vi "Ic Distribution_box.vi"(0 "device in":tag="Dev1", 1 "Scale factor":dbl=1.0, 2 "maximum value":dbl=5.0 format="%#_13g", 3 "Log Data":bool=TRUE, 5 "Trigger source":tag="/Dev1/PFI0", 7 "Current Read":tag="Dev1/ai2", 9 "Sample Rate":dbl=50.0 format="%.3p", 11 "error in no error":errorcluster, 12 "Points Number":i32=10000, 13 "Points per loop":i32=1000, 14 "minimum value":dbl format="%#_13g") -> (4 "Ic array":dbl[](array[numeric]), 15 "error out":errorcluster)   [LabVIEW 2021]
uses:
  <vilib>/DAQmx/read.llb/DAQmx Read (Analog 1D DBL 1Chan NSamp).vi
  <vilib>/DAQmx/create/channels.llb/DAQmx Create Channel (AI-Voltage-Basic).vi
  <vilib>/DAQmx/configure/timing.llb/DAQmx Timing (Sample Clock).vi
  <vilib>/DAQmx/miscellaneous.llb/DAQmx Fill In Error Info.vi
  Transport measurement/VIs/global.vi
  <vilib>/Analysis/NI_AALBase.lvlib
panel:
  out "millisecond timer value":u32=9828879
  in  "Tab Control":enum32{"AWG", "DAQ", "Curve", "Error"}(tab)=enum."Curve"
  in  "Sampling Frequency Hz":u64=10000000
  in  "End time S":dbl=0.005
  in  "Delay time S":dbl=0.3
  in  "Ramp time S":dbl=0.01
  in  "Amplitude V":dbl=5.0 format="%#_13g"
  in  "Channel Name":u16(ring)=1 items=["1"=1, "2"=2, "3"=3, "4"=4]
  in  "Update Wave":bool=TRUE
  in  "Use AWG":bool
  out "Points get":i32=10000
  in  "intervals":i32=100
  out "Histogram Graph":T1(graph)={"X Values"=[3.5826407117095322, 3.586252819563783, 3.589864927418034, 3.5934770352722847, 3.5970891431265355, 3.6007012509807863, 3.604313358835037, 3.607925466689288, 3.6115375745435387, 3.6151496823977896, 3.6187617902520404, 3.622373898106291, 3.625986005960542, 3.629598113814793, 3.6332102216690436, 3.6368223295232944, 3.6404344373775452, 3.644046545231796, 3.647658653086047, 3.6512707609402977, 3.6548828687945485, 3.6584949766487993, 3.66210708450305, 3.665719192357301, 3.6693313002115517, 3.6729434080658026, 3.6765555159200534, 3.680167623774304, 3.683779731628555, 3.687391839482806, 3.6910039473370566, 3.6946160551913074, 3.6982281630455582, 3.701840270899809, 3.70545237875406, 3.7090644866083107, 3.7126765944625615, 3.7162887023168123, 3.719900810171063, 3.723512918025314, 3.7271250258795647, 3.7307371337338155, 3.7343492415880664, 3.737961349442317, 3.741573457296568, 3.745185565150819, 3.7487976730050696, 3.7524097808593204, 3.7560218887135712, 3.759633996567822, 3.763246104422073, 3.7668582122763237, 3.7704703201305745, 3.7740824279848253, 3.777694535839076, 3.781306643693327, 3.7849187515475777, 3.7885308594018285, 3.7921429672560794, 3.79575507511033, 3.799367182964581, 3.802979290818832, 3.8065913986730826, 3.8102035065273334, 3.8138156143815842, 3.817427722235835, 3.821039830090086, 3.8246519379443367, 3.8282640457985875, 3.8318761536528383, 3.835488261507089, 3.83910036936134, 3.8427124772155907, 3.8463245850698415, 3.8499366929240924, 3.853548800778343, 3.857160908632594, 3.860773016486845, 3.8643851243410956, 3.8679972321953464, 3.8716093400495972, 3.875221447903848, 3.878833555758099, 3.8824456636123497, 3.8860577714666005, 3.8896698793208513, 3.893281987175102, 3.896894095029353, 3.9005062028836037, 3.9041183107378545, 3.9077304185921053, 3.911342526446356, 3.914954634300607, 3.918566742154858, 3.9221788500091086, 3.9257909578633594, 3.92940306571761, 3.933015173571861, 3.936627281426112, 3.9402393892803627], "Histogram: h(x)"=[1, 2, 1, 1, 1, 3, 7, 5, 7, 6, 7, 7, 16, 15, 14, 11, 15, 15, 23, 24, 29, 23, 38, 51, 47, 57, 64, 70, 75, 78, 87, 101, 101, 122, 128, 134, 149, 157, 181, 164, 172, 179, 223, 221, 232, 234, 241, 277, 236, 272, 250, 272, 270, 306, 299, 280, 265, 274, 270, 255, 244, 229, 218, 223, 211, 204, 190, 153, 135, 142, 127, 128, 102, 96, 75, 79, 57, 44, 43, 39, 33, 25, 21, 26, 13, 19, 20, 10, 9, 2, 2, 2, 5, 2, 1, 2, 2, 1, 0, 1]}
  in  "stop":bool
  # "Voltage read by DAQ times Scale factor= Ic in uA"
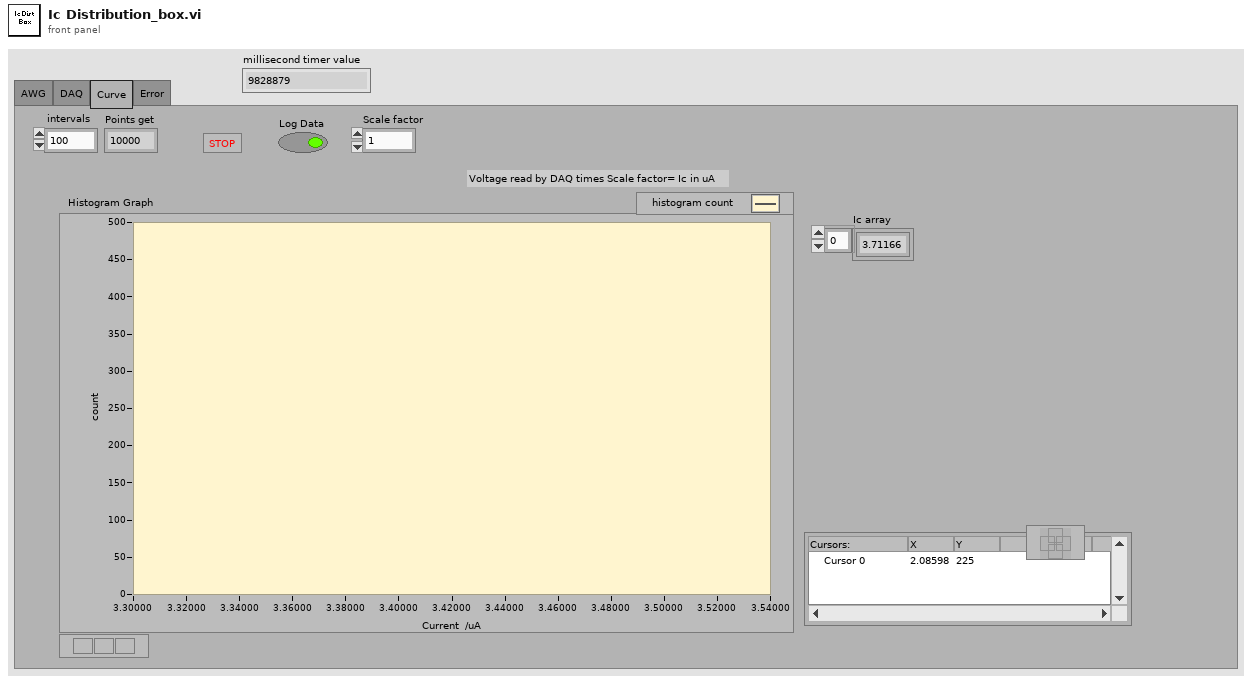
[diagram p1: front panel]
types:
  T1 = cluster{"X Values":dbl[], "Histogram: h(x)":i32[]}
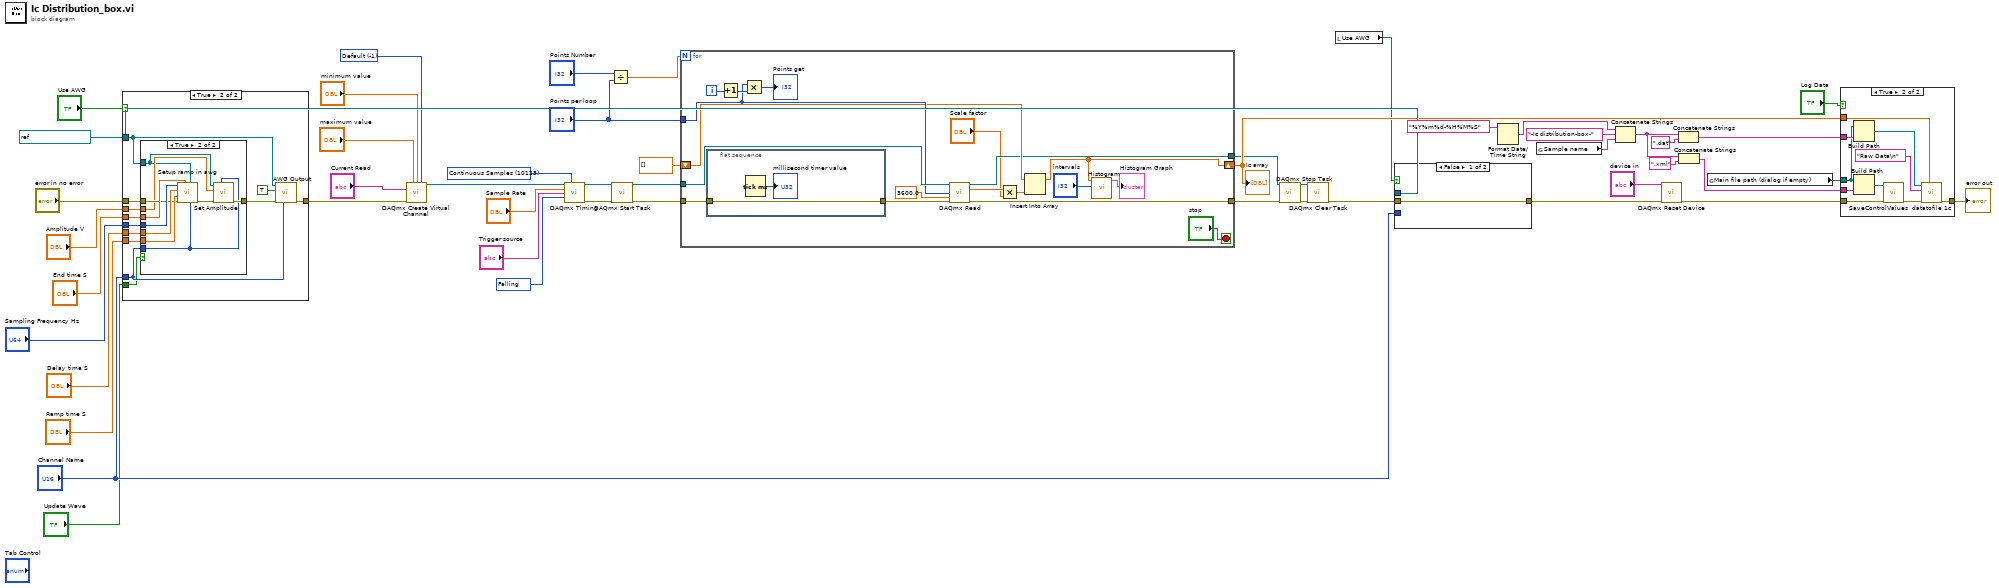
[diagram p0: block diagram]
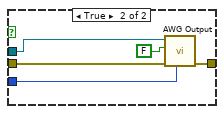
[diagram p3: hidden frame]
diagram:
  w42 = refnum<visa-resource-name> "GPIB0::1::INSTR" ("VISA resource name")
  w16 = 10171 items=["Rising"=10280, "Falling"=10171] ("active edge")
  w17 = 10123 items=["Finite Samples"=10178, "Continuous Samples"=10123, "Hardware Timed Single Point"=12522] ("sample mode")
  w22 = -1 items=["Default"=-1, "RSE"=10083, "NRSE"=10078, "Differential"=10106, "Pseudodifferential"=12529] ("input terminal configuration")
  n1 = case shown="True" "Use AWG" {
    tunnel: "Sampling Frequency Hz" -> [_ w63]
    tunnel: "End time S" -> [_ w62]
    tunnel: "Delay time S" -> [_ w61]
    tunnel: "Ramp time S" -> [_ w60]
    tunnel: "error in no error" -> [w51 w59]
    tunnel: "Amplitude V" -> [_ w58]
    tunnel: "Channel Name" -> [_ w57]
    tunnel: w42 -> [_ w56]
    tunnel: "Update Wave" -> [_ w55]
    tunnel: [w51 w54] -> w21
    frame False {
    }
    frame True {
      n2 = case shown="True" w55 {
        tunnel: w63 -> [_ w74]
        tunnel: w62 -> [_ w73]
        tunnel: w61 -> [_ w72]
        tunnel: w60 -> [_ w71]
        tunnel: w59 -> [w64 w70]
        tunnel: w58 -> [_ w69]
        tunnel: [w64 w67] -> w53
        tunnel: w57 -> [_ w66]
        tunnel: w56 -> [_ w65]
        frame False {
        }
        frame True {
          n3 = call "Setup ramp in awg.vi"("Channel Name (1)"=w66, "VISA resource name"=w65, "End time S"=w73, "error in (no error)"=w70, "Ramp time S"=w71, "Delay time S"=w72, "Sampling Frequency (Hz)"=w74) -> ("error out"=w68:errorcluster)  [unwired: 4 in]
          n4 = call "Set Amplitude.vi"("Channel Name (1)"=w66, "error in (no error)"=w68, "Amplitude V"=w69, "VISA resource name"=w65) -> ("error out"=w67:errorcluster)  [unwired: 7 in]
        }
      }
      n5 = call "AWG Output.vi"("Channel Name (1)"=w57, "error in (no error)"=w53, "Enable Output (T: Enable)"=TRUE, "VISA resource name"=w56) -> ("error out"=w54:errorcluster)  [unwired: 7 in]
    }
  }
  n6 = call-poly <vilib>:"DAQmx Create Virtual Channel.vi"("maximum value"="maximum value", "minimum value"="minimum value", "input terminal configuration"=w22, "physical channels"="Current Read", "error in"=w21) -> ("task out"=w20:refnum<k21>)  [unwired: 9 in, 1 out]
  n7 = call-poly <vilib>:"DAQmx Timing.vi"("task/channels in"=w20, "sample mode"=w17, "rate"="Sample Rate", "source"="Trigger source", "active edge"=w16) -> ("task out"=w15:refnum<k21>, "error out"=w14:errorcluster)  [unwired: 9 in]
  n8 = Divide(x="Points Number", y="Points per loop") -> (x/y=w12:dbl)
  n9 = call <vilib>:"DAQmx Start Task.vi"("task/channels in"=w15, "error in"=w14) -> ("task out"=w10:refnum<k21>, "error out"=w9:errorcluster)  [unwired: 12 in]
  n10 = for {
    N: w12 -> [_]
    shift-right: [w82] -> w27
    shift-left: dbl[] [] -> [w83]
    tunnel: [w81] -> w6
    tunnel: "Points per loop" -> [w84]
    tunnel: w10 -> [w86]
    tunnel: w9 -> [w76]
    tunnel: [w80] -> w4
    i -> [w92]
    stop <- "stop" stop-if-true
    n11 = flat-sequence {
      tunnel: w76 -> [w94]
      tunnel: [w94] -> w75
      frame #0 {
        n12 = Tick Count (ms)() -> (millisecond timer value=→"millisecond timer value":u32)
      }
    }
    n13 = Increment(x=w92) -> (x+1=w88:i32)
    n14 = Multiply(x=w84, y=w88) -> (x*y=→"Points get":i32)
    n15 = call-poly <vilib>:"DAQmx Read.vi"("task/channels in"=w86, "number of samples per channel"=w84, "timeout"=3600.0, "error in"=w75) -> ("task out"=w80:refnum<k21>, "data"=w79:dbl[], "error out"=w81:errorcluster)  [unwired: 9 in]
    n16 = Multiply(x=w79, y="Scale factor") -> (x*y=w77:dbl[])
    n17 = Insert Into Array(array=w83, new element=w77) -> (w82:dbl[])  [unwired: 1 in]
    n18 = call <vilib>:"Histogram.vi"("intervals"="intervals", "X"=w82) -> ("Histogram Graph"=→"Histogram Graph":T1)  [unwired: 6 in, 3 out]
  }
  "Ic array" <- w27
  n19 = call <vilib>:"DAQmx Stop Task.vi"("task/channels in"=w4, "error in"=w6) -> ("task out"=w8:refnum<k21>, "error out"=w7:errorcluster)  [unwired: 12 in]
  n20 = call <vilib>:"DAQmx Clear Task.vi"("task in"=w8, "error in"=w7) -> ("error out"=w5:errorcluster)  [unwired: 13 in]
  n21 = local read "Use AWG"() -> (w2:bool)
  n22 = case shown="False" w2 {
    tunnel: "Channel Name" -> [_ w100]
    tunnel: w42 -> [_ w99]
    tunnel: [w95 w98] -> w41
    tunnel: w5 -> [w95 w97]
    frame False {
    }
    frame True {
      n23 = call "AWG Output.vi"("Channel Name (1)"=w100, "error in (no error)"=w97, "Enable Output (T: Enable)"=FALSE, "VISA resource name"=w99) -> ("error out"=w98:errorcluster)  [unwired: 7 in]
    }
  }
  n24 = Format Date/Time String(time format string (%c)="%Y%m%d-%H%M%S") -> (date/time string=w37:string)  [unwired: 2 in]
  n25 = global read "global.vi" "Sample name"() -> (w35:string)
  n26 = Concatenate Strings(w37, "-Ic distribution-box-" ("string"), w35) -> (w32:string)
  n27 = call <vilib>:"DAQmx Reset Device.vi"("device in"="device in", "error in"=w41) -> ("error out"=w28:errorcluster)  [unwired: 13 in]
  n28 = Concatenate Strings(w32, ".dat" ("string")) -> (w33:string)
  n29 = Concatenate Strings(w32, ".xml" ("string")) -> (w29:string)
  n30 = global read "global.vi" "Main file path (dialog if empty)"() -> (w30:path)
  n31 = case shown="True" "Log Data" {
    tunnel: w33 -> [_ w110]
    tunnel: w30 -> [_ w109]
    tunnel: w29 -> [_ w108]
    tunnel: w28 -> [w101 w104]
    tunnel: w27 -> [_ w103]
    tunnel: [w101 w102] -> w26
    frame False {
    }
    frame True {
      n32 = Build Path(base path=w109, name or relative path=w110) -> (appended path=w105:path)
      n33 = Build Path(base path=w109, name or relative path=w108) -> (appended path=w107:path)
      n34 = call "SaveControlValues.vi"("XML File Path"=w107, "error in (no error)"=w104) -> ("error out"=w106:errorcluster)  [unwired: 8 in]
      n35 = call "datatofile 1c.vi"("A1"=w103, "error in"=w106, "title"="Raw Data\n", "file path (dialog if empty)"=w105) -> ("error out"=w102:errorcluster)  [unwired: 7 in]
    }
  }
  "error out" <- w26
